vi "clear.vi"(8 "error in (no error)":errorcluster, 11 "DL090216RangeOffsetImageProcessor in":refnum<class "ImageProcessorDL090216RangeOffset.lvclass">) -> (0 "error out":errorcluster, 3 "DL090216RangeOffsetImageProcessor out":refnum<class "ImageProcessorDL090216RangeOffset.lvclass">)   [LabVIEW 2010, in "ImageProcessorDL090216RangeOffset.lvclass"]
uses:
  ImageProcessorDL090216RangeOffset.lvclass
  ImageProcessorDL090216RangeOffset.lvclass/ImageProcessorDL090216RangeOffset.ctl
  GenericImageProcessor/GenericImageProcessor/GenericImageProcessor.lvclass
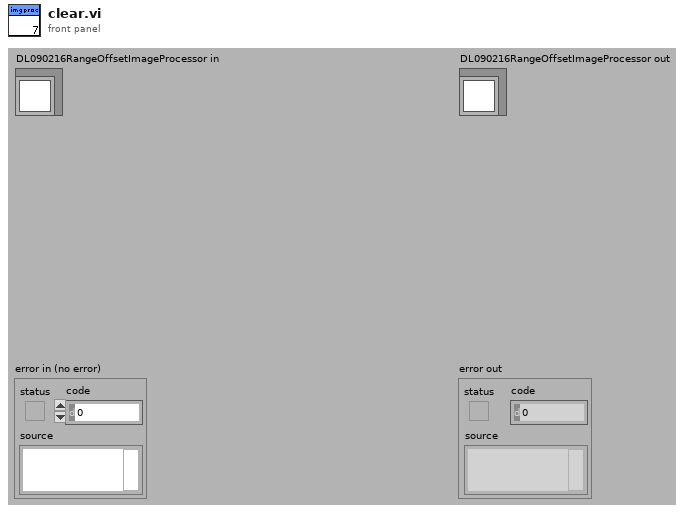
[diagram p1: front panel]
types:
  T1 = typedef "range_offset_cluster.ctl" = cluster{"range":dbl, "offset":dbl}
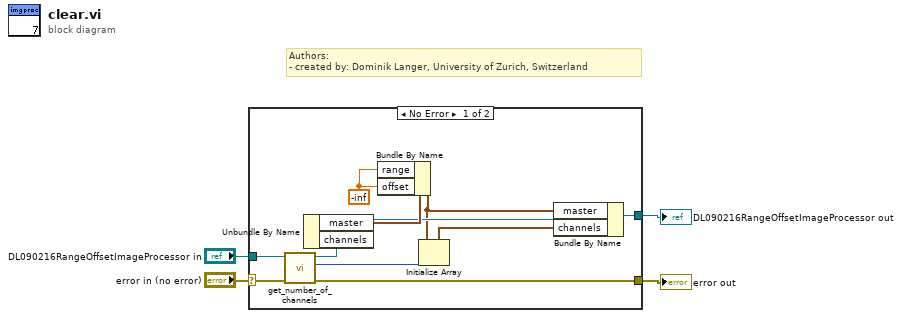
[diagram p0: block diagram]
diagram:
  # "Authors: \n- created by: Dominik Langer, University of Zurich, Switzerland"
  n1 = case shown="No Error" "error in (no error)" {
    selector: "error in (no error)" -> [w11 w16]
    tunnel: [w10 w16] -> w3
    tunnel: [w14 w15] -> w1
    tunnel: "DL090216RangeOffsetImageProcessor in" -> [w9 w15]
    frame No Error {
      w13 = -inf
      n2 = call "get_number_of_channels.vi"("error in (no error)"=w11, "GenericImageProcessor.lvclass in"=w9) -> ("error out"=w10:errorcluster, "number of channels"=w6:i32, "GenericImageProcessor.lvclass out"=w8:refnum<class "ImageProcessorDL090216RangeOffset.lvclass">)  [unwired: 7 out]
      n3 = Unbundle By Name(w8) -> ("master"=w12:T1)  [unwired: 1 out]
      n4 = Bundle By Name(cluster=w12, "range"=w13, "offset"=w13) -> (w7:T1)
      n5 = Initialize Array(w7, w6) -> (w5:T1[])
      n6 = Bundle By Name(cluster=w8, "master"=w7, "channels"=w5) -> (w14:refnum<class "ImageProcessorDL090216RangeOffset.lvclass">)
    }
    frame Error {
    }
  }
  "error out" <- w3
  "DL090216RangeOffsetImageProcessor out" <- w1
